vi "Setup TS.vi"(8 "error in (no error)":errorcluster, 11 "Generic Test Stand in":refnum<class "Generic Test Stand.lvclass">) -> (0 "error out":errorcluster, 3 "Generic Test Stand out":refnum<class "Generic Test Stand.lvclass">)   [LabVIEW 2019, in "Generic Test Stand.lvclass"]
uses:
  Generic Test Stand.lvclass
  Generic Test Stand.lvclass/Generic Test Stand.ctl
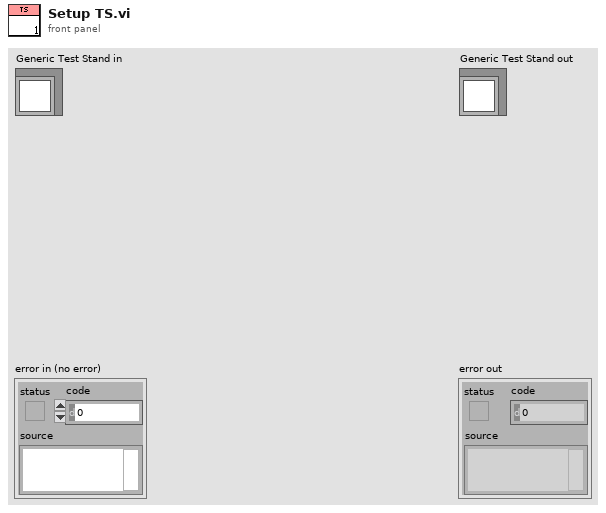
[diagram p1: front panel]
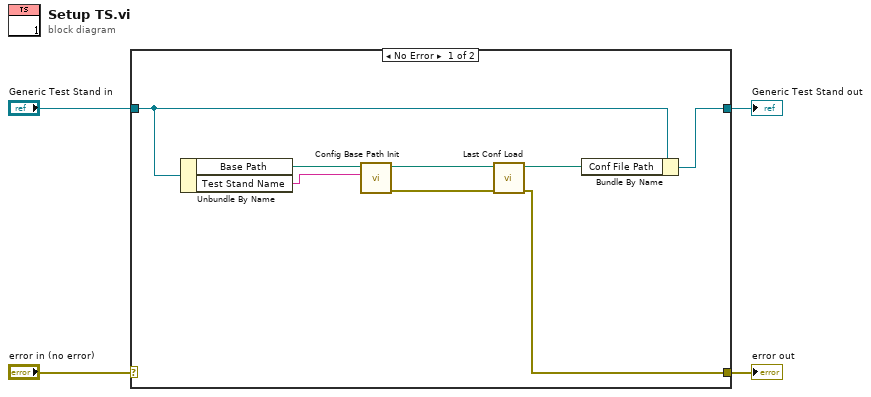
[diagram p0: block diagram]
diagram:
  n1 = case shown="No Error" "error in (no error)" {
    selector: "error in (no error)" -> [_ w14]
    tunnel: [w6 w14] -> w3
    tunnel: [w8 w13] -> w1
    tunnel: "Generic Test Stand in" -> [w11 w13]
    frame No Error {
      n2 = Unbundle By Name(w11) -> ("Base Path"=w10:path, "Test Stand Name"=w9:string)
      n3 = call "Config Base Path Init.vi"("TS Name"=w9, "base path"=w10) -> ("error out"=w5:errorcluster, "TS Config Folder Path"=w12:path)  [unwired: 8 in]
      n4 = call "Last Conf Load.vi"("error in"=w5, "Config Dir"=w12) -> ("error out"=w6:errorcluster, "Conf File path"=w7:path)  [unwired: 8 in]
      n5 = Bundle By Name(cluster=w11, "Conf File Path"=w7) -> (w8:refnum<class "Generic Test Stand.lvclass">)
    }
    frame Error {
    }
  }
  "error out" <- w3
  "Generic Test Stand out" <- w1
